vi "LP_Testing.vi"() -> ()   [LabVIEW 2012]
uses:
  BotSpeakSubs/BotspeakSettingsUsed.vi
  SubVIs/LVPresent_Globals.vi
panel:
  out "Button":bool
  in  "LED5":bool
  in  "LED4":bool
  in  "LED2":bool
  in  "LED3":bool
  in  "LED1":bool
  out "Light":u8(slide) scale=0.0..255.0
  # "Test the LilyPad\n\nTry pushing the button or reading the light sensor.  You can click on any of the areas to see the program that is running"
  # "Move your finger over the sensor to see the bar change!"
  # "Click these to turn on the LEDs!"
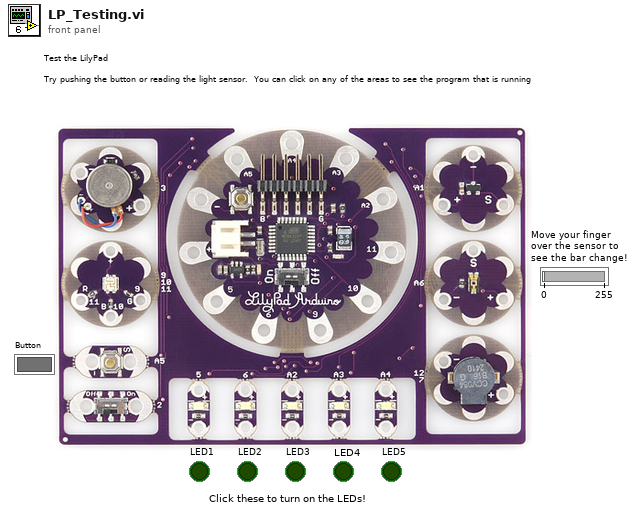
[diagram p1: front panel]
types:
  T1 = typedef "BotSpeak_Control.ctl" = cluster{"Address":string, "Reply EOF":string, "Hardware":string, "Retries":i8, "Timeout":i32}
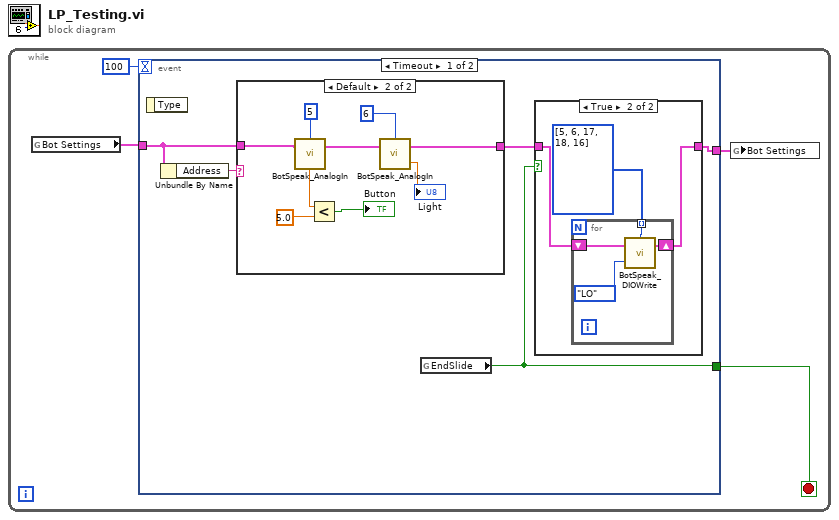
[diagram p0: block diagram]
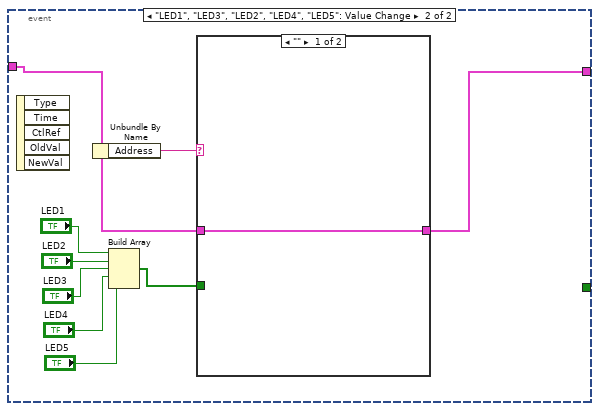
[diagram p4: hidden frame]
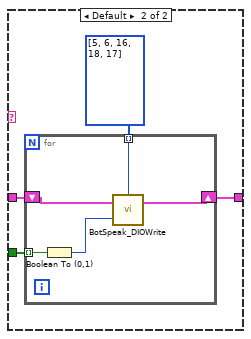
[diagram p5: hidden frame]
diagram:
  n1 = while {
    stop <- w4 stop-if-true
    n2 = global read "BotspeakSettingsUsed.vi" "Bot Settings"() -> (w2:T1)
    n3 = event shown="[0] Timeout" {
      selector: _ -> [_ _]
      dyn-events: _ -> [_ _]
      timeout: 100 -> [_ _]
      tunnel: [w7 _] -> w4
      tunnel: w2 -> [w8 w29]
      tunnel: [w5 w30] -> w1
      event Timeout {
        n4 = event-data() -> ()  [unwired: 1 in, 1 out]
        n5 = Unbundle By Name(w8) -> ("Address"=w9:string)
        n6 = case shown="Default" w9 {
          tunnel: [w18 w26] -> w6
          tunnel: w8 -> [w18 w25]
          frame "" {
          }
          frame Default {
            n7 = call <userlib>:"BotSpeak_AnalogIn.vi"("Bot Settings"=w25, "A/D Channel"=u32 5 ("DIO Line")) -> ("voltage"=w21:dbl, "Bot Settings"=w24:T1)  [unwired: 1 in]
            n8 = Less?(x=w21, y=5.0) -> (x < y?=→"Button":bool)
            n9 = call <userlib>:"BotSpeak_AnalogIn.vi"("Bot Settings"=w24, "A/D Channel"=u8 6) -> ("voltage"=→"Light":dbl, "Bot Settings"=w26:T1)  [unwired: 1 in]
          }
        }
        n10 = global read "LVPresent_Globals.vi" "EndSlide"() -> (w7:bool)
        n11 = case shown="True" w7 {
          tunnel: w6 -> [w10 w12]
          tunnel: [w10 w11] -> w5
          frame False {
          }
          frame True {
            n12 = for {
              tunnel: i32[] [5, 6, 17, 18, 16] -> [w17] mode=indexing
              shift-right: [w14] -> w11
              shift-left: w12 -> [w15]
              n13 = call <userlib>:"BotSpeak_DIOWrite.vi"("State"=enum32{"LO", "HI"}."LO", "Bot Settings"=w15, "DIO Line"=w17) -> ("Bot Settings"=w14:T1)  [unwired: 1 out]
            }
          }
        }
      }
      event "LED1", "LED3", "LED2", "LED4", "LED5": Value Change {
        n14 = event-data() -> ()  [unwired: 1 in, 5 out]
        n15 = Unbundle By Name(w29) -> ("Address"=w28:string)
        n16 = Build Array("LED1", "LED2", "LED3", "LED4", "LED5") -> (w31:bool[])
        n17 = case shown="\"\"" w28 {
          tunnel: w31 -> [_ w40]
          tunnel: w29 -> [w37 w39]
          tunnel: [w37 w38] -> w30
          frame "" {
          }
          frame Default {
            n18 = for {
              tunnel: i32[] [5, 6, 16, 18, 17] ("Array") -> [w45] mode=indexing
              tunnel: w40 -> [w44] mode=indexing
              shift-right: [w42] -> w38
              shift-left: w39 -> [w43]
              n19 = Boolean To (0,1)(Boolean=w44) -> (0, 1=w46:i16)
              n20 = call <userlib>:"BotSpeak_DIOWrite.vi"("State"=w46, "Bot Settings"=w43, "DIO Line"=w45) -> ("Bot Settings"=w42:T1)  [unwired: 1 out]
            }
          }
        }
      }
    }
    n21 = global write "BotspeakSettingsUsed.vi" "Bot Settings"(w1) -> ()
  }
